vi "test at_bt_status_0.vi"() -> ()   [LabVIEW 2012]
panel:
  out "numer \niteracji":i32
  in  "ilosc iteracji":i32
  out "close error":errorcluster
  out "incoming \ndata table":string[](array[string])
  out "data out":string
  out "read error":errorcluster
  out "write error":errorcluster
  out "open error":errorcluster
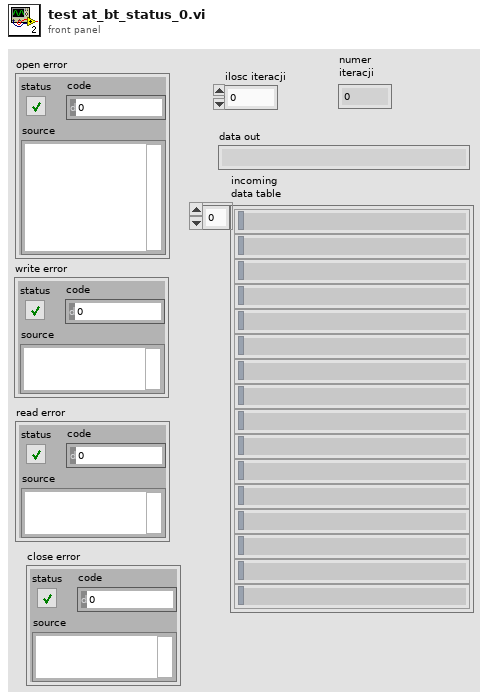
[diagram p1: front panel]
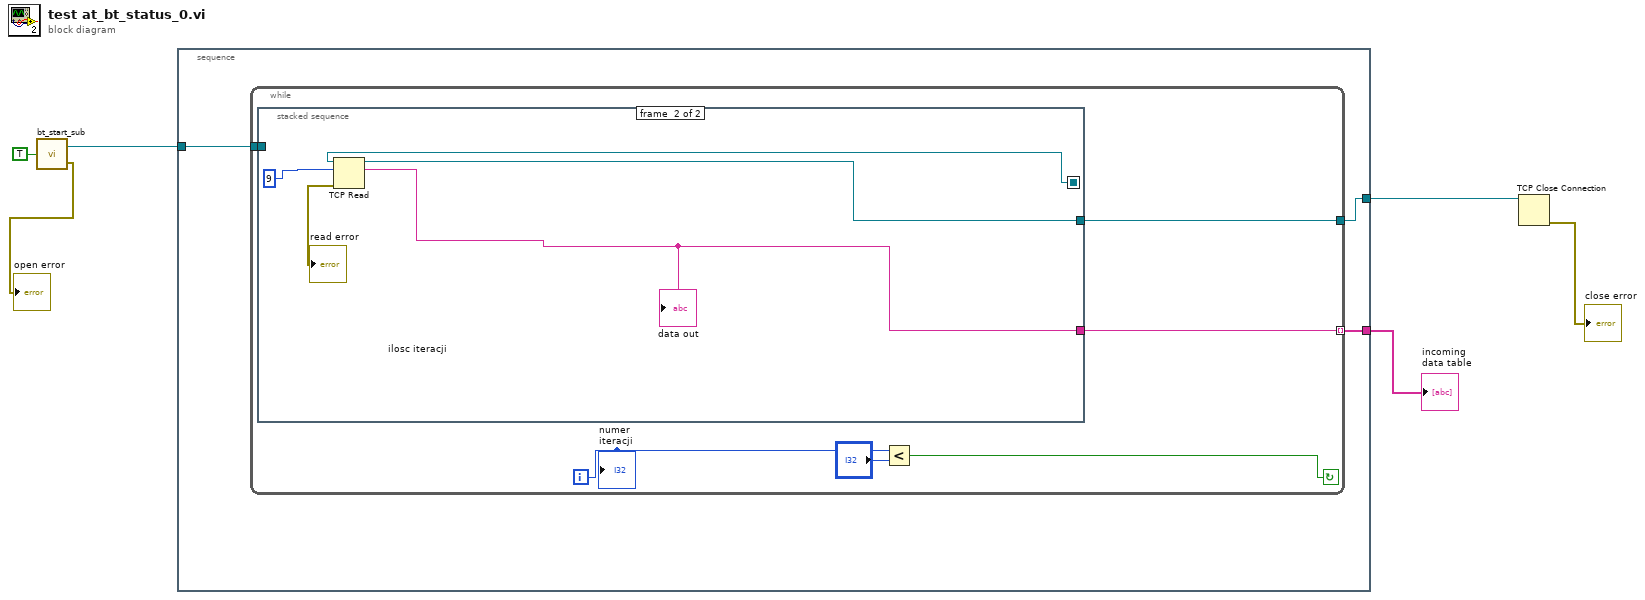
[diagram p0: block diagram]
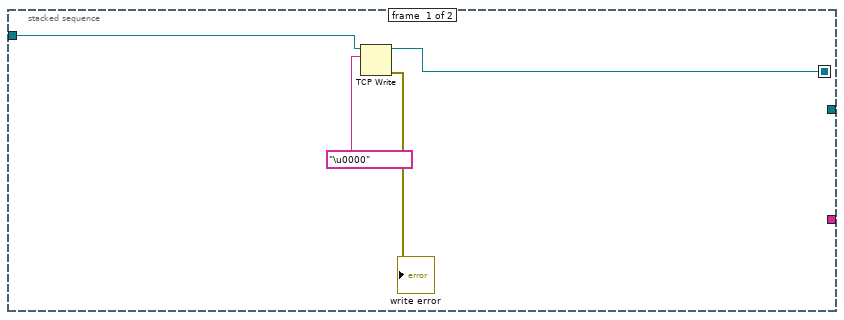
[diagram p2: hidden frame]
diagram:
  n1 = call "bt_start_sub.vi"("auto?"=TRUE) -> ("connection ID"=w5:refnum<k31>, "open error"=→"open error":errorcluster)
  n2 = stacked-sequence {
    tunnel: w5 -> [w9]
    tunnel: [w8] -> w4
    tunnel: [w7] -> w3
    frame #0 {
      n3 = while {
        tunnel: w9 -> [w15]
        tunnel: [w11] -> w8
        tunnel: [w10] -> w7 mode=indexing
        i -> [w14]
        stop <- w12 continue-if-true
        n4 = stacked-sequence {
          seq-local: [w16 _] -> [_ w22]
          tunnel: w15 -> [w19 _]
          tunnel: [_ w21] -> w11
          tunnel: [_ w20] -> w10
          frame #0 {
            n5 = TCP Write(connection ID=w19, data in="\u0000") -> (connection ID out=w16:refnum<k31>, error out=→"write error":errorcluster)  [unwired: 2 in, 1 out]
          }
          frame #1 {
            n6 = TCP Read(connection ID=w22, bytes to read=9) -> (connection ID out=w21:refnum<k31>, data out=w20:string, error out=→"read error":errorcluster)  [unwired: 3 in]
            "data out" <- w20
          }
        }
        n7 = Less?(x=w14, y="ilosc iteracji") -> (x < y?=w12:bool)
        "numer \niteracji" <- w14
      }
    }
  }
  "incoming \ndata table" <- w3
  n8 = TCP Close Connection(connection ID=w4) -> (error out=→"close error":errorcluster)  [unwired: 2 in, 1 out]
